vi "_026.vi"(11 "Celsius":dbl) -> (3 "Farenhiet":dbl)   [LabVIEW 2024]
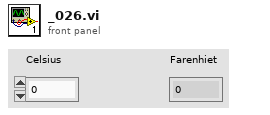
[diagram p1: front panel]
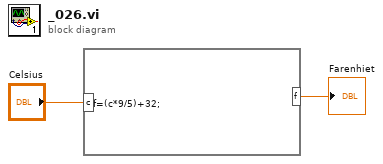
[diagram p0: block diagram]
diagram:
  n1 = formula code="f=(c*9/5)+32;"("c"="Celsius") -> ("f"=→"Farenhiet":dbl)
